vi "End stop control-Steffen’s MacBook Pro.vi"(0 "Threshold Lower":dbl=3025.0, 1 "t":bool, 3 "Bor - Frequency [Hz]":dbl, 4 "output cluster":T26 {"A/SPI - LiDAR"."SPI Configuration"."Frame Length" min=1 max=16}, 5 "Min (ms puls bredde)":dbl, 6 "error in (no error)":errorcluster, 8 "Threshold Upper":dbl=3175.0, 9 "Max (ms puls bredde)":dbl, 13 "Bor - Duty Cycle":dbl) -> (14 "Grounded?":bool, 15 "Output Dutycycle \nPWM":dbl, 16 "ALL BOTTOM":bool, 17 "Bottom Array":bool[](array[boolean]), 20 "Within Drill limits?":bool, 21 "ALL TOP":bool, 22 "Move Only?":bool, 24 "Movement Output":T27(ring), 25 "HOLD":bool, 26 "error out":errorcluster, 27 "Top Array":bool[](array[boolean]))   [LabVIEW 2018]
uses:
  <vilib>/myRIO/Instrument Drivers/Onboard IO/DIO/typedefs/DIO Reference.ctl
  <vilib>/myRIO/Common/Instrument Driver Framework/Utilities/typedefs/myRIO Generic Hardware Reference.ctl
  <vilib>/myRIO/Common/Instrument Driver Framework/Utilities/typedefs/Hardware Version Enum.ctl
  <vilib>/myRIO/Common/Instrument Driver Framework/Utilities/typedefs/myRIO v1.0 Reference.ctl
  <vilib>/myRIO/Common/Instrument Driver Framework/Utilities/typedefs/Generic FPGA Reference.ctl
  <vilib>/myRIO/Common/Instrument Driver Framework/myRIO v1.0/DIO/typedefs/DIO Channels List.ctl
  <vilib>/myRIO/Common/Instrument Driver Framework/myRIO v1.0/DIO/typedefs/DIO Channels Enum.ctl
  <vilib>/myRIO/Instrument Drivers/Onboard IO/PWM/typedefs/PWM Reference.ctl
  <vilib>/myRIO/Common/Instrument Driver Framework/myRIO v1.0/PWM/typedefs/PWM Channels Enum.ctl
  <vilib>/myRIO/Instrument Drivers/Onboard IO/PWM/typedefs/PWM Configuration.ctl
  <vilib>/myRIO/Instrument Drivers/Onboard Devices/Accelerometer/typedefs/Accelerometer Reference.ctl
  <vilib>/myRIO/Common/Instrument Driver Framework/myRIO v1.0/Accelerometer/typedefs/Accelerometer Channels List.ctl
  <vilib>/myRIO/Common/Instrument Driver Framework/myRIO v1.0/Accelerometer/typedefs/Accelerometer Channels Enum.ctl
  <vilib>/myRIO/Instrument Drivers/Onboard IO/AI/typedefs/AI Reference.ctl
  <vilib>/myRIO/Common/Instrument Driver Framework/myRIO v1.0/AI/typedefs/AI Channels List.ctl
  <vilib>/myRIO/Common/Instrument Driver Framework/myRIO v1.0/AI/typedefs/AI Channels Enum.ctl
  <vilib>/myRIO/Common/Instrument Driver Framework/Utilities/typedefs/Analog Scaling Constants List.ctl
  <vilib>/myRIO/Common/Instrument Driver Framework/Utilities/typedefs/Analog Scaling Constants.ctl
  <vilib>/myRIO/Instrument Drivers/Onboard IO/SPI/typedefs/SPI Reference.ctl
  <vilib>/myRIO/Common/Instrument Driver Framework/myRIO v1.0/SPI/typedefs/SPI Channels Enum.ctl
  <vilib>/myRIO/Instrument Drivers/Onboard IO/SPI/typedefs/SPI Configuration.ctl
  <vilib>/myRIO/Common/Instrument Driver Framework/myRIO v1.0/SPI/typedefs/SPI Clock Phase.ctl
  <vilib>/myRIO/Common/Instrument Driver Framework/myRIO v1.0/SPI/typedefs/SPI Clock Polarity.ctl
  <vilib>/myRIO/Common/Instrument Driver Framework/myRIO v1.0/SPI/typedefs/SPI Data Direction.ctl
  <vilib>/myRIO/Common/Instrument Driver Framework/myRIO v1.0/SPI/typedefs/SPI Frame Length.ctl
  <vilib>/Utility/error.llb/Error Cluster From Error Code.vi
  <vilib>/myRIO/Common/Instrument Driver Framework/myRIO v1.0/DIO/vis/myRIO v1.0 Read DIO.vi
  <vilib>/myRIO/Instrument Drivers/Onboard IO/DIO/DIO.lvlib
  <vilib>/myRIO/Instrument Drivers/Onboard IO/PWM/PWM.lvlib
  <vilib>/myRIO/Instrument Drivers/Onboard Devices/Accelerometer/Accelerometer.lvlib
  <vilib>/myRIO/Instrument Drivers/Onboard IO/AI/AI.lvlib
  <vilib>/myRIO/Instrument Drivers/Onboard IO/SPI/SPI.lvlib
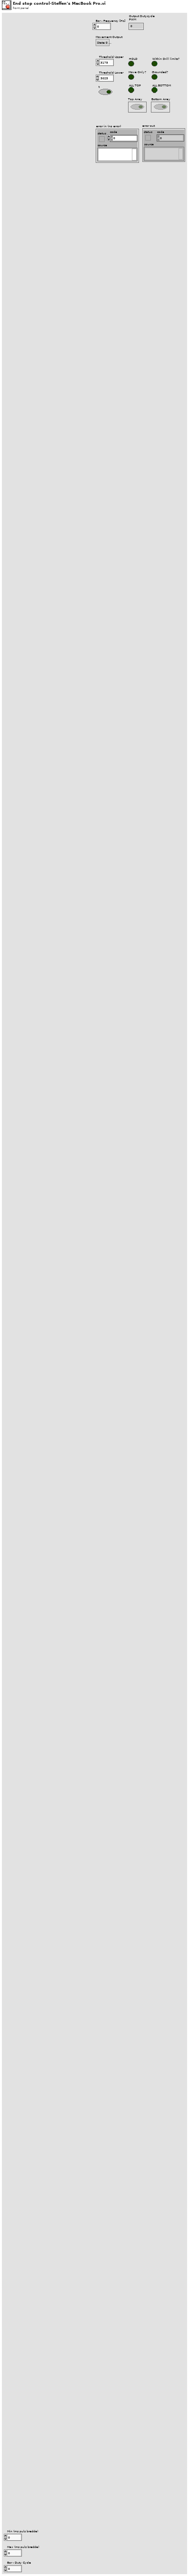
[diagram p1: front panel]
types:
  T1 = typedef "DIO.lvlib/DIO Reference.ctl" = cluster{"myRIO Reference":T2, "DIO Channels List":T6}
  T2 = typedef "myRIO Generic Hardware Reference.ctl" = cluster{"myRIO Model":T3, "myRIO Hardware Reference":T4}
  T3 = typedef "Hardware Version Enum.ctl" = enum16{"Unknown", "myRIO-1900", "myRIO-1950", "roboRIO", "NI ELVIS RIO CM", "ELVIS III"}
  T4 = typedef "myRIO v1.0 Reference.ctl" = cluster{"Generic FPGA Reference":T5, "Allow multiple opens":bool}
  T5 = typedef "Generic FPGA Reference.ctl" = refnum<k20>
  T6 = typedef "DIO Channels List.ctl" = T7[]
  T7 = typedef "DIO Channels Enum.ctl" = enum16{"Not Connected", "C/DIO0", "C/DIO1", "C/DIO2", "C/DIO3", "C/DIO4", "C/DIO5", "C/DIO6", "C/DIO7", "A/DIO0", "A/DIO1", "A/DIO2", "A/DIO3", "A/DIO4", "A/DIO5", "A/DIO6", "A/DIO7", "A/DIO8", "A/DIO9", "A/DIO10", "A/DIO11", "A/DIO12", "A/DIO13", "A/DIO14", "A/DIO15", "A/DIO16", "A/DIO17", "A/DIO18", "A/DIO19", "B/DIO0", "B/DIO1", "B/DIO2", "B/DIO3", "B/DIO4", "B/DIO5", "B/DIO6", "B/DIO7", "B/DIO8", "B/DIO9", "B/DIO10", "B/DIO11", "B/DIO12", "B/DIO13", "B/DIO14", "B/DIO15", "B/DIO16", "B/DIO17", "B/DIO18", "B/DIO19", "LED0", "LED1", "LED2", "LED3", "Button0", "DIO/DIO0", "DIO/DIO1", "DIO/DIO2", "DIO/DIO3", "DIO/DIO4", "DIO/DIO5", "DIO/DIO6", "DIO/DIO7", "DIO/DIO8", "DIO/DIO9", "SPI/CS0", "SPI/CS1", "SPI/CS2", "SPI/CS3", "LED RADIO (Green)", "LED RADIO (Red)", "LED COMM (Green)", "LED COMM (Red)", "LED MODE (Green)", "LED MODE (Red)"}
  T8 = typedef "PWM.lvlib/PWM Reference.ctl" = cluster{"myRIO Reference":T2, "PWM Channels Enum":T9, "PWM Configuration":T10}
  T9 = typedef "PWM Channels Enum.ctl" = enum16{"Not Connected", "C/PWM0", "C/PWM1", "A/PWM0", "A/PWM1", "A/PWM2", "A/PWM3", "A/PWM4", "A/PWM5", "A/PWM6", "A/PWM7", "A/PWM8", "A/PWM9", "A/PWM10", "A/PWM11", "A/PWM12", "A/PWM13", "A/PWM14", "A/PWM15", "A/PWM16", "A/PWM17", "A/PWM18", "A/PWM19", "B/PWM0", "B/PWM1", "B/PWM2", "B/PWM3", "B/PWM4", "B/PWM5", "B/PWM6", "B/PWM7", "B/PWM8", "B/PWM9", "B/PWM10", "B/PWM11", "B/PWM12", "B/PWM13", "B/PWM14", "B/PWM15", "B/PWM16", "B/PWM17", "B/PWM18", "B/PWM19", "PWM/PWM0", "PWM/PWM1", "PWM/PWM2", "PWM/PWM3", "PWM/PWM4", "PWM/PWM5", "PWM/PWM6", "PWM/PWM7", "PWM/PWM8", "PWM/PWM9"}
  T10 = typedef "PWM.lvlib/PWM Configuration.ctl" = cluster{"Frequency":dbl, "Duty Cycle":dbl}
  T11 = typedef "Accelerometer.lvlib/Accelerometer Reference.ctl" = cluster{"myRIO Reference":T2, "Accelerometer Channels List":T12, "LSB Weight":dbl}
  T12 = typedef "Accelerometer Channels List.ctl" = T13[]
  T13 = typedef "Accelerometer Channels Enum.ctl" = enum16{"Not Connected", "X-Axis", "Y-Axis", "Z-Axis"}
  T14 = typedef "AI.lvlib/AI Reference.ctl" = cluster{"myRIO Reference":T2, "AI Channels List":T15, "AI Scaling Constants List":T17}
  T15 = typedef "AI Channels List.ctl" = T16[]
  T16 = typedef "AI Channels Enum.ctl" = enum16{"Not Connected", "AudioIn/Left", "AudioIn/Right", "C/AI0", "C/AI1", "A/AI0", "A/AI1", "A/AI2", "A/AI3", "A/AI4", "A/AI5", "A/AI6", "A/AI7", "B/AI0", "B/AI1", "B/AI2", "B/AI3", "B/AI4", "B/AI5", "B/AI6", "B/AI7", "AI/AI0", "AI/AI1", "AI/AI2", "AI/AI3", "A/AI0 (DIFF)", "A/AI1 (DIFF)", "A/AI2 (DIFF)", "A/AI3 (DIFF)", "B/AI0 (DIFF)", "B/AI1 (DIFF)", "B/AI2 (DIFF)", "B/AI3 (DIFF)"}
  T17 = typedef "Analog Scaling Constants List.ctl" = T18[]
  T18 = typedef "Analog Scaling Constants.ctl" = cluster{"LSB Weight (Volts)":dbl, "Offset (Volts)":dbl, "Signed?":bool}
  T19 = typedef "SPI.lvlib/SPI Reference.ctl" = cluster{"myRIO Reference":T2, "SPI Channels Enum":T20, "SPI Configuration":T21}
  T20 = typedef "SPI Channels Enum.ctl" = enum16{"Not Connected", "A/SPI", "B/SPI", "SPI/SPI"}
  T21 = typedef "SPI.lvlib/SPI Configuration.ctl" = cluster{"Frequency [Hz]":dbl, "Clock Phase":T22, "Clock Polarity":T23, "Data Direction":T24, "Frame Length":T25}
  T22 = typedef "SPI Clock Phase.ctl" = enum8{"Leading", "Trailing"}
  T23 = typedef "SPI Clock Polarity.ctl" = enum8{"Low", "High"}
  T24 = typedef "SPI Data Direction.ctl" = enum8{"Most significant bit first", "Least significant bit first"}
  T25 = typedef "SPI Frame Length.ctl" = u8
  T26 = cluster{"B/DIO0 - Stepper Direction":T1, "B/DIO1 - Stepper1 Enable":T1, "B/DIO2 - Stepper2 Enable":T1, "B/DIO3 - Stepper3 Enable":T1, "B/DIO4 - Endstop Stepper1 Top":T1, "B/DIO11 - Endstop Stepper1 Bund":T1, "B/DIO12 - Endstop Stepper2 Top":T1, "B/DIO13 - Endstop Stepper2 Bund":T1, "B/DIO14 - Endstop Stepper3 Top":T1, "B/DIO15 - Endstop Stepper3 Bund":T1, "A/DIO0 - Cooler":T1, "A/DIO1 - Beacon drop (dio1)":T1, "A/DIO2 - Beacon drop (dio0)":T1, "A/DIO3 - QuickRelease (dio1)":T1, "A/DIO4 - QuickRelease (dio0)":T1, "A/DIO11 - LiDAR SPI CS":T1, "B/PWM0 - Stepper":T8, "B/PWM1 - Drill":T8, "A/PWM0 - Servo_Roll":T8, "A/PWM1 - Servo_Yaw":T8, "Acc. X-axis":T11, "Acc. Y-axis":T11, "B/AI0 - Drone Grounded F3":T14, "B/AI1 - Drone Drill Gear F4":T14, "B/AI2 - Beacon Drop F5":T14, "B/AI3 - Drone Drill Boost F6":T14, "A/AI0 - Drone Stepper F8":T14, "A/AI1 - Beacon Wiper":T14, "A/AI2 - QuickRelease Wiper":T14, "A/AI3 - Drill Current":T14, "A/SPI - LiDAR":T19, "B/UART - XBee":refnum<visa-resource-name>, "A/UART - A3 GPS":refnum<visa-resource-name>, "RIO Flashing LEDs":T1}
  T27 = enum16{"State 0 - Default", "State 1 - Go down", "State 2 - Go up", "State 3 - Triangle Wobble"}
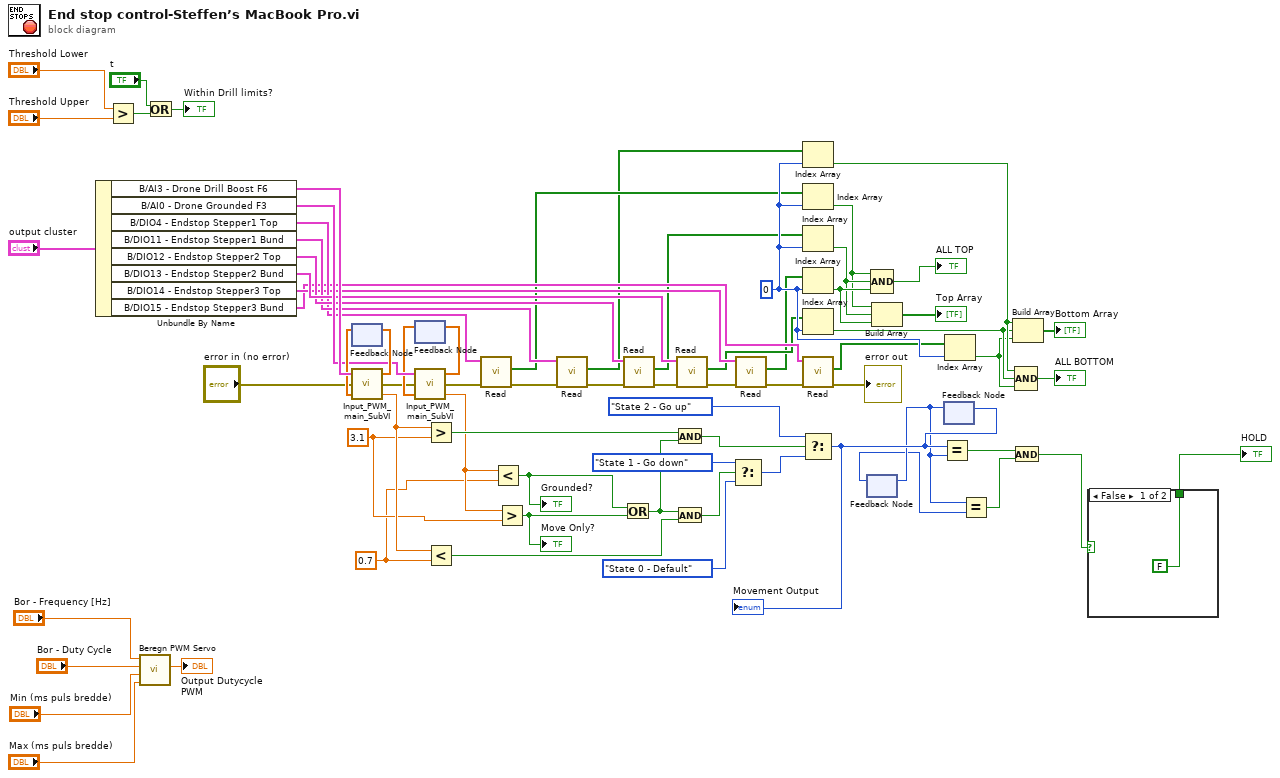
[diagram p0: block diagram]
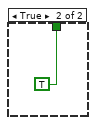
[diagram p2: hidden frame]
diagram:
  w4 = 0.7 ("y")
  w5 = 3.1 ("y")
  w35 = 0 ("index")
  n1 = Unbundle By Name("output cluster") -> ("B/AI3 - Drone Drill Boost F6"=w58:T14, "B/AI0 - Drone Grounded F3"=w55:T14, "B/DIO4 - Endstop Stepper1 Top"=w49:T1, "B/DIO11 - Endstop Stepper1 Bund"=w50:T1, "B/DIO12 - Endstop Stepper2 Top"=w51:T1, "B/DIO13 - Endstop Stepper2 Bund"=w52:T1, "B/DIO14 - Endstop Stepper3 Top"=w48:T1, "B/DIO15 - Endstop Stepper3 Bund"=w47:T1)
  n2 = Greater?(x="Threshold Lower", y="Threshold Upper") -> (0:w44:bool)
  n3 = call "Beregn PWM Servo.vi"("Max (ms puls bredde)"="Max (ms puls bredde)", "Min (ms puls bredde)"="Min (ms puls bredde)", "Duty Cycle"="Bor - Duty Cycle", "Frekvens"="Bor - Frequency [Hz]") -> ("Output Dutycycle til PWM Servo"=→"Output Dutycycle \nPWM":dbl)  [unwired: 7 in]
  n4 = Or(x="t", y=w44) -> (x .or. y?=→"Within Drill limits?":bool)
  n5 = feedback #1() -> (w57:dbl[])  [unwired: 1 in]
  n6 = call "Input_PWM_main_SubVI.vi"("Shift in"=w57, "error in (no error)"="error in (no error)", "AI Ref In"=w58) -> ("Value out"=w62:dbl, "error out"=w18:errorcluster, "Shift out"=w56:dbl[])
  n7 = feedback-in #1(w56) -> ()
  n8 = feedback #2() -> (w54:dbl[])  [unwired: 1 in]
  n9 = call "Input_PWM_main_SubVI.vi"("Shift in"=w54, "error in (no error)"=w18, "AI Ref In"=w55) -> ("Value out"=w9:dbl, "error out"=w17:errorcluster, "Shift out"=w19:dbl[])
  n10 = feedback-in #2(w19) -> ()
  n11 = Greater?(x=w62, y=w5) -> (0:w67:bool)
  n12 = Less?(x=w62, y=w4) -> (x < y?=w66:bool)
  n13 = call <vilib>:"Read.vi"("error in (no error)"=w17, "DIO Ref In"=w49) -> ("error out"=w16:errorcluster, "Values"=w34:bool[])  [unwired: 7 in, 1 out]
  n14 = Less?(x=w9, y=w4) -> (x < y?=w8:bool)
  "Grounded?" <- w8
  n15 = Greater?(x=w9, y=w5) -> (0:w6:bool)
  "Move Only?" <- w6
  n16 = call <vilib>:"Read.vi"("error in (no error)"=w16, "DIO Ref In"=w50) -> ("error out"=w15:errorcluster, "Values"=w33:bool[])  [unwired: 7 in, 1 out]
  n17 = Or(x=w8, y=w6) -> (x .or. y?=w7:bool)
  n18 = call <vilib>:"Read.vi"("error in (no error)"=w15, "DIO Ref In"=w51) -> ("error out"=w14:errorcluster, "Values"=w32:bool[])  [unwired: 7 in, 1 out]
  n19 = And(x=w67, y=w7) -> (x .and. y?=w63:bool)
  n20 = And(x=w7, y=w66) -> (x .and. y?=w59:bool)
  n21 = call <vilib>:"Read.vi"("error in (no error)"=w14, "DIO Ref In"=w52) -> ("error out"=w13:errorcluster, "Values"=w31:bool[])  [unwired: 7 in, 1 out]
  n22 = Select(t=T27."State 1 - Go down" ("Enum"), s=w59, f=T27."State 0 - Default" ("Enum")) -> (s? t:f=w65:T27)
  n23 = call <vilib>:"Read.vi"("error in (no error)"=w13, "DIO Ref In"=w48) -> ("error out"=w12:errorcluster, "Values"=w30:bool[])  [unwired: 7 in, 1 out]
  n24 = Index Array(array=w33, index=w35) -> (element=w24:bool)
  n25 = Index Array(array=w34, index=w35) -> (element=w38:bool)
  n26 = Index Array(array=w32, index=w35) -> (element=w39:bool)
  n27 = Index Array(array=w30, index=w35) -> (element=w40:bool)
  n28 = Index Array(array=w31, index=w35) -> (element=w23:bool)
  n29 = call <vilib>:"Read.vi"("error in (no error)"=w12, "DIO Ref In"=w47) -> ("error out"=→"error out":errorcluster, "Values"=w29:bool[])  [unwired: 7 in, 1 out]
  n30 = Select(t=T27."State 2 - Go up" ("Enum"), s=w63, f=w65) -> (s? t:f=w71:T27)
  "Movement Output" <- w71
  n31 = feedback #3() -> (w2:T27)  [unwired: 1 in]
  n32 = Compound Arithmetic op=AND(w38, w39, w40) -> (→"ALL TOP":bool)
  n33 = Build Array(w38, w39, w40) -> (→"Top Array":bool[])
  n34 = feedback #4() -> (w68:T27)  [unwired: 1 in]
  n35 = feedback-in #3(w68) -> ()
  n36 = Equal?(x=w71, y=w68) -> (x = y?=w70:bool)
  n37 = feedback-in #4(w71) -> ()
  n38 = Index Array(array=w29, index=w35) -> (element=w22:bool)
  n39 = Equal?(x=w68, y=w2) -> (x = y?=w69:bool)
  n40 = And(x=w70, y=w69) -> (x .and. y?=w1:bool)
  n41 = Build Array(w24, w23, w22) -> (→"Bottom Array":bool[])
  n42 = Compound Arithmetic op=AND(w24, w23, w22) -> (→"ALL BOTTOM":bool)
  n43 = case shown="False" w1 {
    tunnel: [FALSE TRUE] -> w3
    frame False {
    }
    frame True {
    }
  }
  "HOLD" <- w3
